vi "Get Spectrum.vi"(8 "error in (no error)":errorcluster, 10 "Channel":u8, 11 "Micron Hyperion Driver in":refnum<class "Micron Hyperion Driver.lvclass">) -> (0 "error out":errorcluster, 2 "Spectrum Graph":cluster{dbl[], "Spectrum, db":dbl[]}[](graph), 3 "Micron Hyperion Driver out":refnum<class "Micron Hyperion Driver.lvclass">)   [LabVIEW 2019, in "Micron Hyperion Driver.lvclass"]
uses:
  Micron Hyperion Driver.lvclass
  C:/GitHub/NHMFL_Core/Libraries/Instruments/Micron Optics/Micron Optics Driver/Micron Optics Driver.lvclass
  Micron Optics Driver/Read Micron Configuration.vi
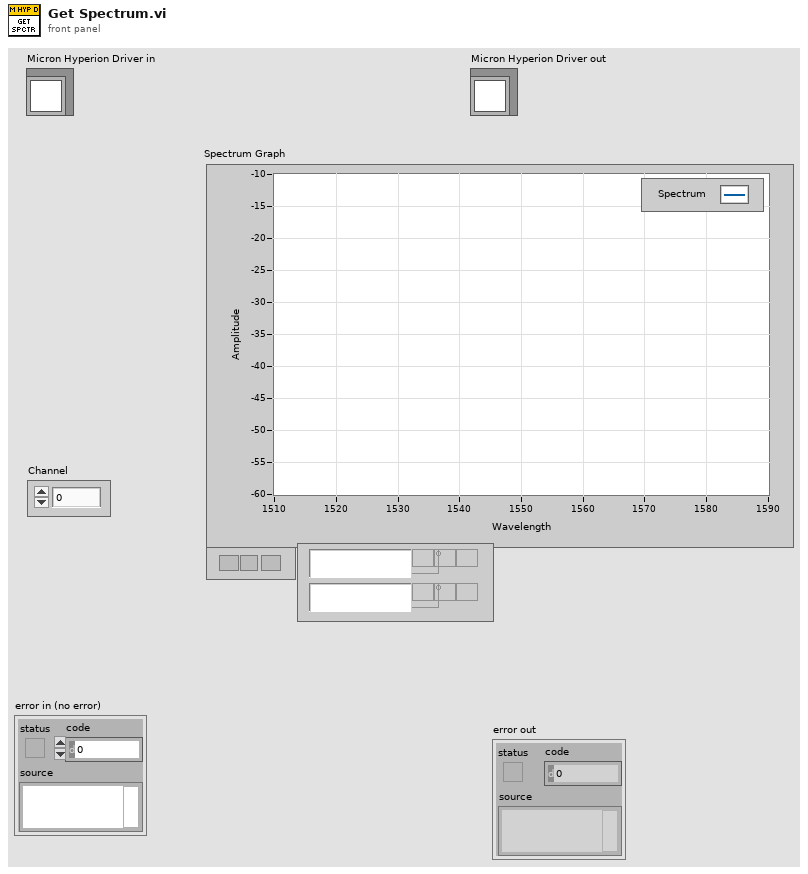
[diagram p1: front panel]
types:
  T1 = typedef "Micron optics configuration.ctl" = cluster{"Reference channel":i32, "Detection Setting IDs":u8[], "Address":string, "Stream and average":bool}
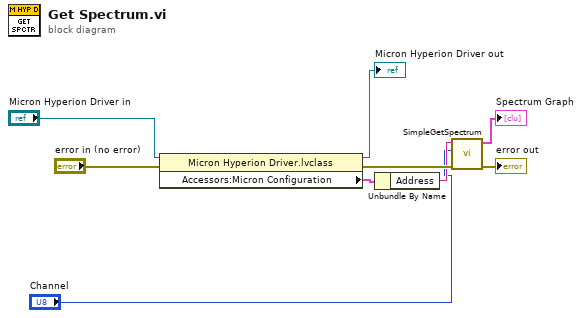
[diagram p0: block diagram]
diagram:
  n1 = property class="Micron Hyperion Driver.lvclass"(reference="Micron Hyperion Driver in", error in="error in (no error)") -> (reference out=→"Micron Hyperion Driver out":refnum<class "Micron Hyperion Driver.lvclass">, error out=w5:errorcluster, "Accessors:Micron Configuration"=w6:T1)
  n2 = Unbundle By Name(w6) -> ("Address"=w2:string)
  n3 = call "SimpleGetSpectrum.vi"("Error In"=w5, "Channel"="Channel", "Address"=w2) -> ("Error Out"=→"error out":errorcluster, "Spectrum Graph"=→"Spectrum Graph":cluster{dbl[], "Spectrum, db":dbl[]}[])  [unwired: 5 in, 2 out]
